vi "WriteTilesToFPGA.vi"(8 "error in (no error)":errorcluster, 9 "Index":u16[](array[numeric]), 10 "Tilecode":u16[](array[numeric]), 11 "Game in":refnum<class "Game.lvclass">) -> (0 "error out":errorcluster, 3 "Game out":refnum<class "Game.lvclass">)   [LabVIEW 2019, in "RT_Game.lvlib" / "Game.lvclass"]
uses:
  Game.lvclass
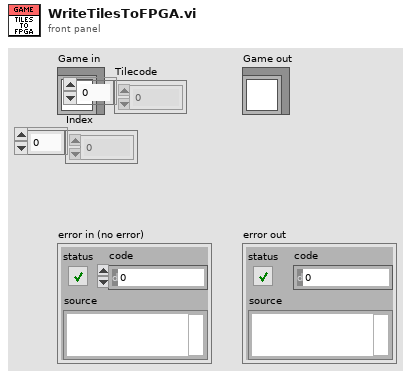
[diagram p1: front panel]
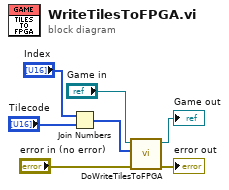
[diagram p0: block diagram]
diagram:
  n1 = Join Numbers(hi="Index", lo="Tilecode") -> ((hi.lo)=w1:u32[])
  n2 = call "DoWriteTilesToFPGA.vi"("error in (no error)"="error in (no error)", "Array"=w1, "Game in"="Game in") -> ("error out"=→"error out":errorcluster, "Game out"=→"Game out":refnum<class "Game.lvclass">)  [unwired: 7 in]
